vi "DAQNavi Create Channel(CI-UpDown Count Value).vi"(0 "task in":i32=-1, 1 "reset times by index":string="-2", 5 "physical channels":string="PCI-1784,BID#0/cntr0", 7 "signal counting type":string(combo)="Omit", 9 "initial value":string="-1", 11 "error in (no error)":errorcluster, 12 "high period":dbl=-1.0, 13 "low period":dbl=-1.0) -> (4 "task out":i32, 15 "error out":errorcluster)   [LabVIEW 2020]
uses:
  DAQNavi_LV.dll
panel:
  in  "pulse width 2":cluster{"high period":dbl, "low period":dbl}
  # "For PCI-1784, the only avaiable initial values are : 0 or 8000000H."
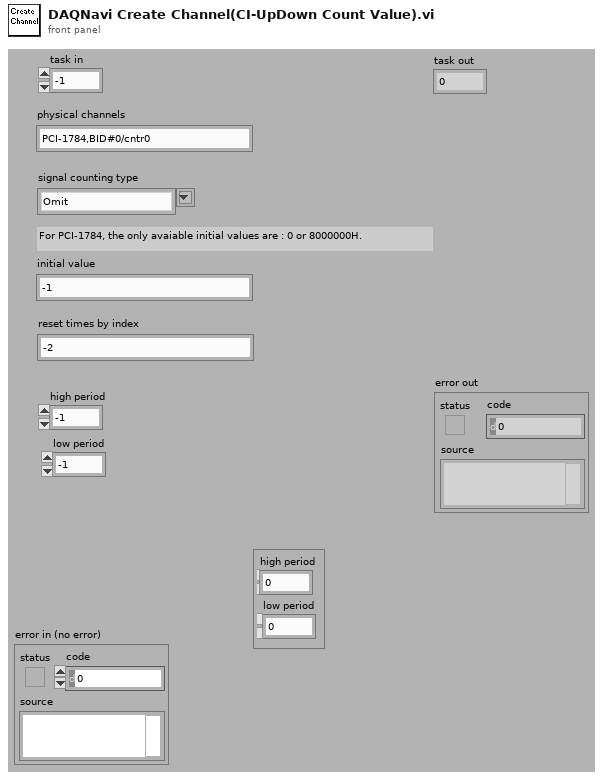
[diagram p1: front panel]
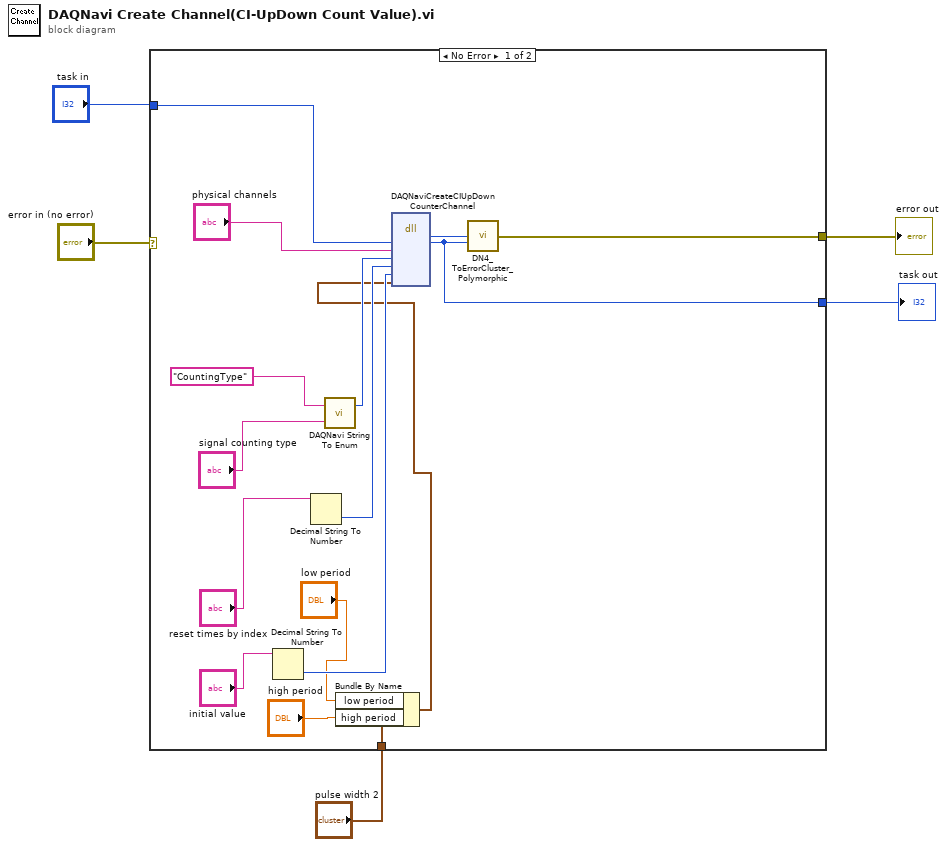
[diagram p0: block diagram]
diagram:
  n1 = case shown="No Error" "error in (no error)" {
    selector: "error in (no error)" -> [_ w22]
    tunnel: "task in" -> [w21 w23]
    tunnel: [w11 w22] -> w3
    tunnel: [w10 w23] -> w2
    tunnel: "pulse width 2" -> [w9 _]
    frame No Error {
      n2 = Decimal String To Number(string="initial value") -> (number=w12:i32)  [unwired: 3 out]
      n3 = Decimal String To Number(string="reset times by index") -> (number=w14:i32)  [unwired: 3 out]
      n4 = call "DAQNavi String To Enum.vi"("enumString"="signal counting type", "enumTypeName"="CountingType") -> ("enumValue"=w16:i32)  [unwired: 1 out]
      n5 = Bundle By Name(cluster=w9, "low period"="low period", "high period"="high period") -> (w6:cluster{"high period":dbl, "low period":dbl})
      n6 = dll-call lib="DAQNavi_LV.dll" fn="DAQNaviCreateCIUpDownCounterChannel"("taskID"=w21, "physicalChannel"="physical channels", "type"=w16, "times"=w14, "initialValue"=w12, "pulseWidth"=w6) -> ("return type"=w19:i32, "taskID"=w10:i32)  [unwired: 8 in, 2 out]
      n7 = call "DN4_ToErrorCluster_Polymorphic.vi"("task id"=w10, "error code"=w19) -> ("error out"=w11:errorcluster)  [unwired: 3 out]
    }
    frame Error {
    }
  }
  "error out" <- w3
  "task out" <- w2
